vi "LVPortGetProperty.vi"(0 "pID":string, 7 "BaseNamepathSrc":string, 9 "Value Type (Or value to update)":variant, 11 "Skip Parent Name (f)":bool, 12 "BaseNamepathSrcAr":string[](array[string])) -> (4 "Value":variant, 8 "Object Map Out":T1[](array[typedef]))   [LabVIEW 2017]
uses:
  Common/ObjectMap/LVPortObjectMapNamepathData.ctl
  Common/ObjectMap/LVPortObjectMapDataTypeEnum.ctl
  Common/ObjectMap/LVPortObjectMapContainerTypeEnum.ctl
  Common/ObjectMap/LVPortObjectMapDefaultIDsEnum.ctl
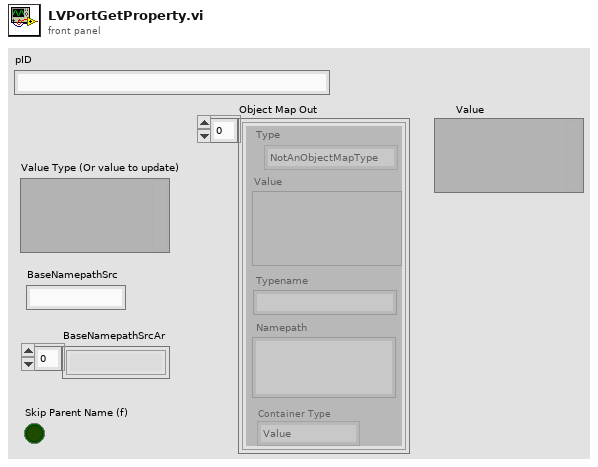
[diagram p1: front panel]
types:
  T1 = typedef "LVPortObjectMapNamepathData.ctl" = cluster{"Type":T2, "Value":variant, "Namepath":string, "Typename":string, "Container Type":T3}
  T2 = typedef "LVPortObjectMapDataTypeEnum.ctl" = enum16{"NotAnObjectMapType", "Real", "Complex", "String", "Boolean"}
  T3 = typedef "LVPortObjectMapContainerTypeEnum.ctl" = enum16{"Value", "Array", "Waveform"}
  T4 = typedef "LVPortObjectMapDefaultIDsEnum.ctl" = i32
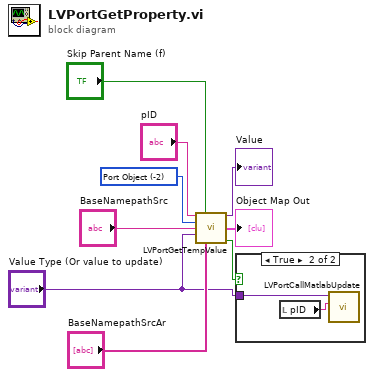
[diagram p0: block diagram]
diagram:
  w8 = T4 -2 items=["No ID"=-1, "Port Object"=-2] ("Default IDs")
  n1 = call "LVPortGetTempValue.vi"("pID"="pID", "Skip Parent Name (t)"="Skip Parent Name (f)", "Object ID"=w8, "BaseNamepathSrc"="BaseNamepathSrc", "Value Type (Or value to update)"="Value Type (Or value to update)", "BaseNamepathSrcAr"="BaseNamepathSrcAr") -> ("Value"=→"Value":variant, "Object Map Out"=→"Object Map Out":T1[], "Has Invalid Indexing or errored value"=w2:bool)  [unwired: 7 in]
  n2 = case shown="True" w2 {
    tunnel: "Value Type (Or value to update)" -> [_ w10]
    frame False {
    }
    frame True {
      n3 = local read "pID"() -> (w11:string)
      n4 = call "LVPortCallMatlabUpdate.vi"("pID"=w11, "Value Type (Or value to update)"=w10) -> ()  [unwired: 10 in]
    }
  }
